vi "UNLOADING_PLAN_UPDATE.vi"(8 "error in (no error)":errorcluster, 10 "SCAN CODE:":string, 11 "Unloading cyc Data in":T1) -> (0 "error out":errorcluster, 2 "QR Match ?":bool, 3 "Unloading cyc Data out":T1)   [LabVIEW 2017]
uses:
  Controls/Unloading_Cyc_Data.ctl
  <vilib>/Utility/file.llb/Read Delimited Spreadsheet (string).vi
  <vilib>/Utility/file.llb/Write Delimited Spreadsheet (string).vi
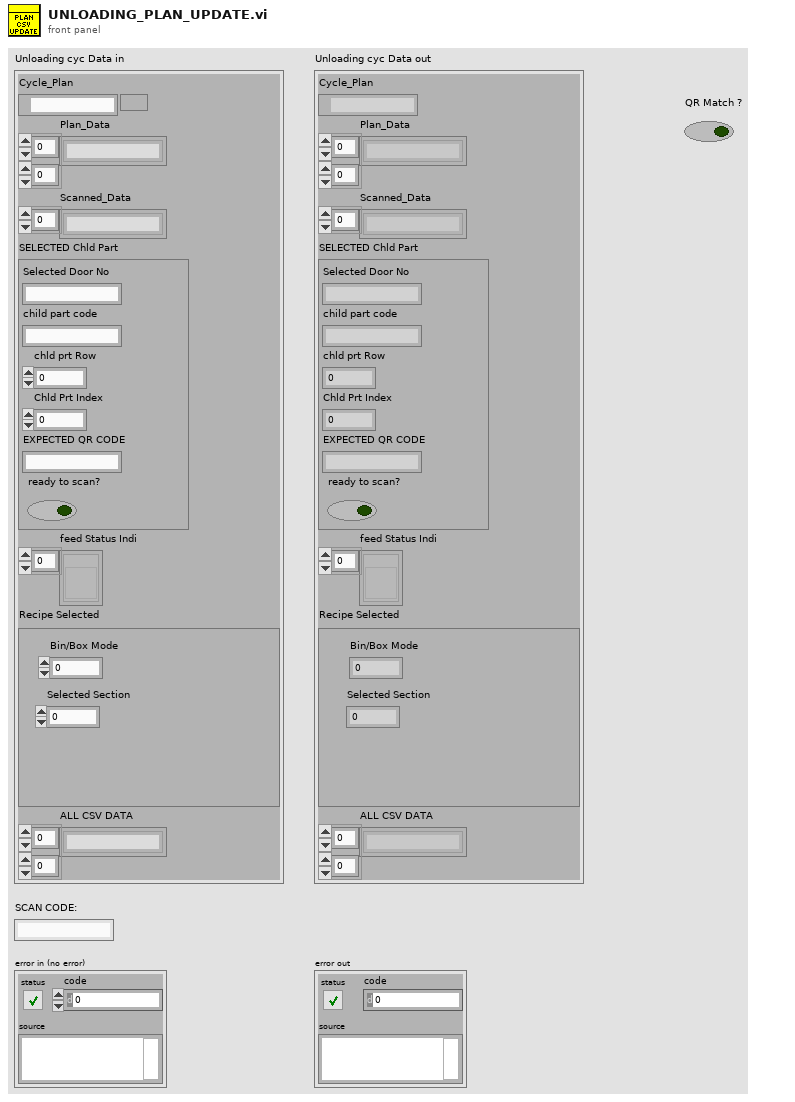
[diagram p1: front panel]
types:
  T1 = typedef "Unloading_Cyc_Data.ctl" = cluster{"Cycle_Plan":path, "Plan_Data":string[][], "Scanned_Data":string[], "SELECTED Chld Part":cluster{"Selected Door No":string, "child part code":string, "chld prt Row":i32, "Chld Prt Index":i32, "EXPECTED QR CODE":string, "ready to scan?":bool}, "feed Status Indi":refnum<vi>[], "Recipe Selected":cluster{"Bin/Box Mode":i32, "Selected Section":i32}, "ALL CSV DATA":string[][]}
  T2 = cluster{"Selected Door No":string, "child part code":string, "chld prt Row":i32, "Chld Prt Index":i32, "EXPECTED QR CODE":string, "ready to scan?":bool}
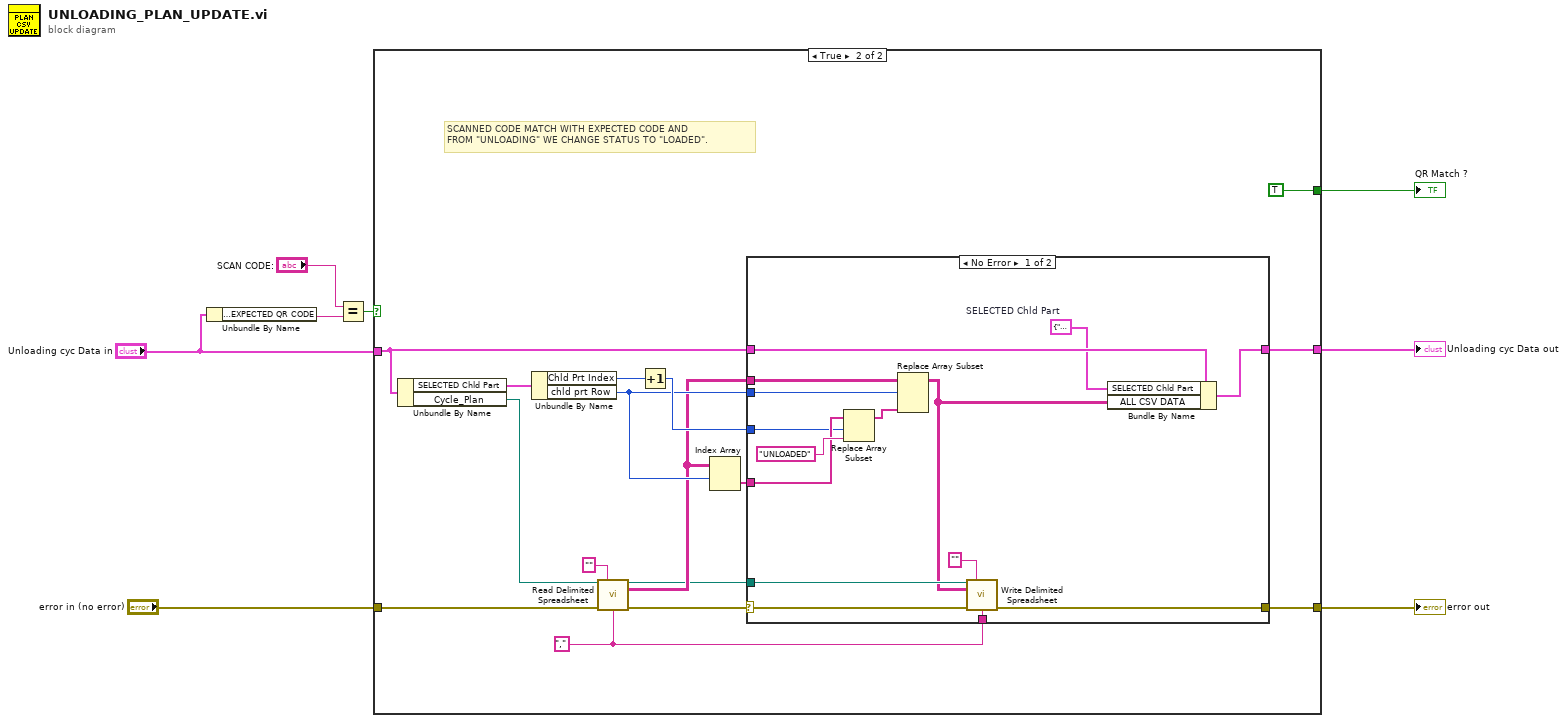
[diagram p0: block diagram]
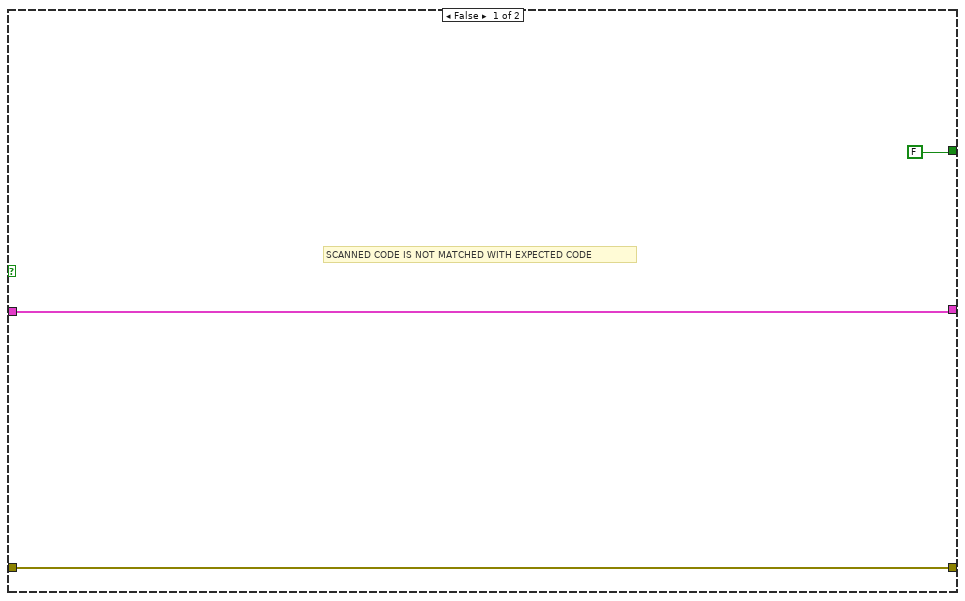
[diagram p2: hidden frame]
diagram:
  n1 = Unbundle By Name("Unloading cyc Data in") -> ("SELECTED Chld Part.EXPECTED QR CODE"=w6:string)
  n2 = Equal?(x="SCAN CODE:", y=w6) -> (x = y?=w8:bool)
  n3 = case shown="True" w8 {
    tunnel: "error in (no error)" -> [w10 w15]
    tunnel: [w10 w16] -> w3
    tunnel: [w11 w13] -> w4
    tunnel: "Unloading cyc Data in" -> [w11 w14]
    tunnel: [FALSE TRUE] -> w1
    frame False {
      # "SCANNED CODE IS NOT MATCHED WITH EXPECTED CODE"
    }
    frame True {
      w18 = ","
      # "SCANNED CODE MATCH WITH EXPECTED CODE AND \nFROM \"UNLOADING\" WE CHANGE STATUS TO \"LOADED\"."
      n4 = Unbundle By Name(w14) -> ("SELECTED Chld Part"=w21:T2, "Cycle_Plan"=w27:path)
      n5 = Unbundle By Name(w21) -> ("Chld Prt Index"=w23:i32, "chld prt Row"=w24:i32)
      n6 = call-poly <vilib>:"Read Delimited Spreadsheet.vi"("file path (dialog if empty)"=w27, "format (%s)"="", "error in (no error)"=w15, "delimiter (\\t)"=w18) -> ("new file path (Not A Path if cancelled)"=w20:path, "all rows"=w22:string[][], "error out"=w19:errorcluster)  [unwired: 6 in, 3 out]
      n7 = Increment(x=w23) -> (x+1=w26:i32)
      n8 = Index Array(array=w22, index (row)=w24) -> (element=w25:string[])  [unwired: 1 in]
      n9 = case shown="No Error" w19 {
        selector: w19 -> [w42 w44]
        tunnel: w20 -> [w41 _]
        tunnel: [w40 w44] -> w16
        tunnel: w22 -> [w39 _]
        tunnel: w18 -> [w36 _]
        tunnel: w24 -> [w35 _]
        tunnel: w25 -> [w34 _]
        tunnel: w26 -> [w30 _]
        tunnel: w14 -> [w32 w43]
        tunnel: [w31 w43] -> w13
        frame No Error {
          w29 = T2 {"Selected Door No"="", "child part code"="", "chld prt Row"=0, "Chld Prt Index"=0, "EXPECTED QR CODE"="", "ready to scan?"=FALSE}  # SELECTED Chld Part
          n10 = Replace Array Subset(array=w34, new element="UNLOADED", index=w30) -> (w37:string[])
          n11 = Replace Array Subset(array=w39, new element=w37, index (row)=w35) -> (w28:string[][])  [unwired: 1 in]
          n12 = call-poly <vilib>:"Write Delimited Spreadsheet.vi"("file path (dialog if empty)"=w41, "format (%s)"="", "2D data"=w28, "error in (no error)"=w42, "delimiter (\\t)"=w36) -> ("error out"=w40:errorcluster)  [unwired: 9 in, 1 out]
          n13 = Bundle By Name(cluster=w32, "SELECTED Chld Part"=w29, "ALL CSV DATA"=w28) -> (w31:T1)
        }
        frame Error {
        }
      }
    }
  }
  "Unloading cyc Data out" <- w4
  "error out" <- w3
  "QR Match ?" <- w1
